vi "Clear Event Module.vi"(7 "Event Module # (1)":u32=1 min=1 max=14, 8 "error in":errorcluster, 9 "Event Module Type (Digital I/O)":T1(ring), 10 "Node In":string, 11 "VISA resource name":refnum<visa-resource-name>) -> (0 "error out":errorcluster, 2 "Node Out":string, 3 "VISA resource name out":refnum<visa-resource-name>, 4 "Command String":string)   [LabVIEW 2009, in "Keithley 2600 Series.lvlib"]
doc: "This VI is used to clear an event module.\n\n<b>Functions and Attributes Used</b>\ndigio.trigger[n].clear()\ntsplink.trigger[n].clear()\nlan.trigger[n].clear()\ntrigger.blender[n].clear()\ntrigger.timer[n].clear()"
uses:
  <instrlib>/Keithley 2600 Series/Keithley 2600 Series.lvlib
  <instrlib>/Keithley 2600 Series/Private/GlobalVariables.vi
panel:
  # "(c) 2008 Keithley Instruments, Inc.  ALL RIGHTS RESERVED."
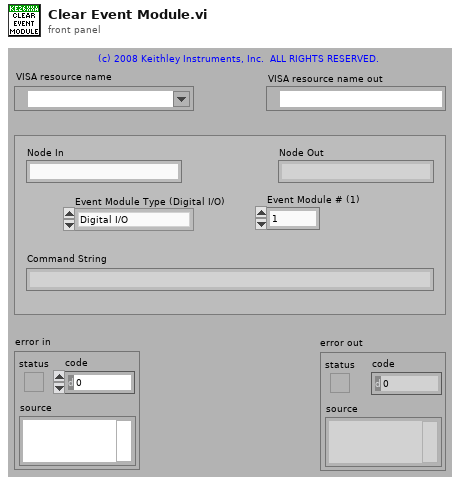
[diagram p1: front panel]
types:
  T1 = enum16{"Digital I/O", "TSP-Link", "LAN", "Blender", "Timer"}
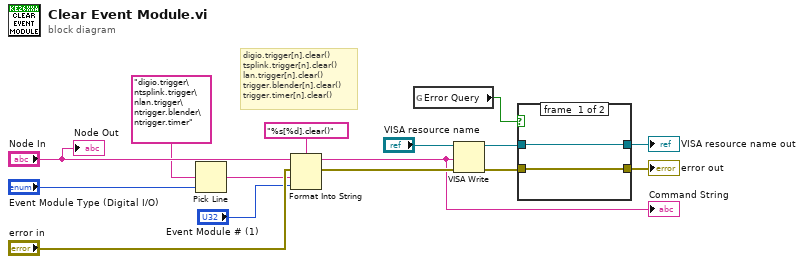
[diagram p0: block diagram]
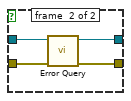
[diagram p2: hidden frame]
diagram:
  # "digio.trigger[n].clear()\ntsplink.trigger[n].clear()\nlan.trigger[n].clear()\ntrigger.blender[n].clear()\ntrigger.timer[n].clear()"
  n1 = Pick Line(multi-line string="digio.trigger\ntsplink.trigger\nlan.trigger\ntrigger.blender\ntrigger.timer", line index="Event Module Type (Digital I/O)") -> (output string=w11:string)  [unwired: 1 out]
  n2 = Format Into String(format string="%s[%d].clear()", initial string="Node In", error in="error in", w11, "Event Module # (1)") -> (resulting string=w4:string, error out=w10:errorcluster)
  "Command String" <- w4
  n3 = global read "GlobalVariables.vi" "Error Query"() -> (w3:bool)
  n4 = VISA Write(VISA resource name="VISA resource name", write buffer=w4, error in (no error)=w10) -> (VISA resource name out=w8:refnum<visa-resource-name>, error out=w7:errorcluster)  [unwired: 1 out]
  n5 = case shown="True" w3 {
    tunnel: w8 -> [w17 w21]
    tunnel: w7 -> [w16 w20]
    tunnel: [w17 w19] -> w6
    tunnel: [w16 w18] -> w5
    frame #0 {
    }
    frame #1 {
      n6 = call <instrlib>:"Error Query.vi"("error in (no error)"=w20, "VISA resource name"=w21) -> ("error out"=w18:errorcluster, "VISA resource name out"=w19:refnum<visa-resource-name>)  [unwired: 8 out]
    }
  }
  "VISA resource name out" <- w6
  "error out" <- w5
  "Node Out" <- "Node In"
